vi "EventLog.Buffer.Reload.vi"(8 "error in":errorcluster, 11 "Path":path) -> (0 "error out":errorcluster, 2 "#loaded entries":i32)   [LabVIEW 2016]
uses:
  EventLog.Buffer.Action.ctl
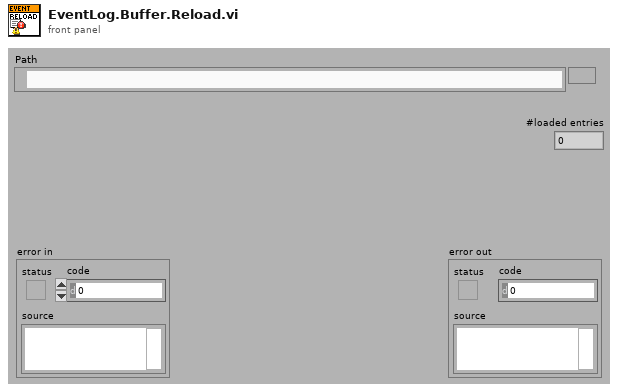
[diagram p1: front panel]
types:
  T1 = typedef "EventLog.Buffer.Action.ctl" = enum16{"init", "re-init", "clear", "set translator", "add", "get", "get unsaved"}
  T2 = typedef "EventLog.Event.ctl" = cluster{"ts":dbl, "lev":T3, "usr":i32, "src":T4, "msg":T5, "arg":variant[]}
  T3 = typedef "EventLog.EventLevel.ctl" = enum8{"Debug", "Info", "Warning", "Error"}
  T4 = typedef "EventLog.EventSource.ctl" = enum16{"All", "Gui", "Ref", "File", "Arch", "Seq", "CPX", "DB", "Laser", "Scan.P", "Scan.O", "PLC"}
  T5 = typedef "Translator.Message.ctl" = enum16{"-", "Event confirmed", "Log out", "Log in", "Shutdown", "Cancel", "Start", "Begin time", "End time", "Duration", "Service Mode", "Ignore Results", "Serial Format", "On", "Off", "OK", "NOK", "NOK %s", "Home", "Work", "Close", "Open", "In progress...", "Missing", "Empty", "Hardware failure", "Initial", "Default", "Total", "Out of range", "Free disk space is below 1GB - contact technician", "Error %d >> %s", "Error %d >> %s >> %s", "Msg %d >> %s", "Laser msg %d %s", "Laser cmd error %s %d", "Laser cmd failed %s", "Laser cmd warning %s", "Laser disconnected", "Laser status %s", "Laser already started", "Laser job unkonwn %s", "Laser job missing %s", "Laser job select failure %s", "Unable to start laser printing (%s)", "Unable to stop laser printing (%s)", "Laser marking aborted", "Laser marking timeout", "Unable to reset Laser Interlock (%s)", "Unable to trigger Laser. Laser not ready (%s)", "Laser job '%s' coordinates not configured", "Starting %s", "Quitting %s", "Configured", "Initializing", "Quitting", "Loading", "Loaded %d results", "Loaded %d events", "Running", "Stopped", "Summary", "Laser", "Do you want to continue?", "Do you want to delete the configuration?", "The configuration is being used by an order. Unable to delete!", "Press confirm button", "Station is not based. Do you want to exit?", "Station requires changeover. Do you want to run the test?", "Test options are not set as default. Do you want to continue?", "Formatting of WabcoNo is disabled. Do you want to continue?", "Product not detected. Do you want to continue?", "Product scan failed. Do you want to continue?", "Calibration", "Log out?", "System", "All", "IDLE", "Translating...%s", "Not found", "Alarm %s", "Run", "Skip", "Abort", "Repeat", "Please wait...", "Database disconnected", "Database disconnected - changeover disabled!", "Login to database successful", "Login to database failed: %d; %s", "Unable to check the product status of reference %d - database disconnected", "Unable to set the product status of reference %d - database disconnected", "Variant file backup %s", "Read variant (%s)", "Result", "Station armed!", "Station requires changeover!", "Select reference number...", "EMERGENCY BUTTON - press Control button", "EMERGENCY DOOR - press Control button", "Resetting Emergency...", "Unable to reset safety circuit - Emergency Button pressed", "Unable to reset safety circuit - Emergency Side Door open", "Station not based", "Station based", "Station not empty", "Station basing...", "No order", "Press Start to begin new order", "Scanning new order", "Order NOK. Correct or scan again", "Order OK. Press Accept", "Order ready", "Revolver incorrect", "Fork incorrect", "Revolver missing", "Revolver empty", "Container missing", "Offline results", "Offline statistics", "Updating statistics %.1f %%", "DMC Configurator", "Door open", "Close the front door", "Press start button", "Done. Open the front door", "Running...", "Running...%.1f %%", "Pause %s", "Pause %s. NOK container missing", "Pause %s. OK container missing", "Pause %s. Revolver empty", "Pause %s. Revolver missing", "Pause %s. Revolver incorrect", "Pause %s. Fork missing", "Pause %s. Fork incorrect", "Pause %s. Too many failures", "Pause %s. Unloading failure", "Pause %s. One slot is not working", "Pause %s. Part order is done. Empty OK container", "Pause %s. Unable to move product to slot", "Pause %s. Unable to move back product pusher", "Pause %s. Unable to lift product", "Pause %s. Unable to move back product lifter", "Pause %s. Unable to move product arm to Work", "Pause %s. Unable to move product arm to NOK", "Pause %s. Unable to move product arm to OK", "Pause %s. Unable to unsuck the NOK product", "Pause %s. Unable to drop the NOK product", "Pause %s. Product OK missing", "Pause %s. Unable to unsuck the OK product", "Pause %s. Unable to drop the OK product", "Stopping...", "File '%s' is missing", "File '%s' is broken", "File '%s' is running", "Log file started (%s)", "Log file ended (%s)", "Log file stopped (%s)", "Log file ignored (%s)", "Log file exported (%s)", "Log file export failed (%s)", "Wrong serial number in log file", "Wrong reference number in log file", "Test steps are missing", "%s = %.3f", "Process param '%s' not found in DB", "Process param '%s' wrong order", "Process param '%s' value %.3f out of limits (%.3f; %.3f)", "Step%d param '%s' not found in DB", "Step%d param '%s' wrong order", "Step%d param '%s' value %.3f out of limits (%.3f; %.3f)", "Step%d EV '%s' not found in DB", "Step%d EV '%s' wrong order", "\"%s\" not found in DB", "\"%s\" wrong order", "\"%s\" value %.3f out of limits (%.3f; %.3f)", "\"%s\" not found in software", "Process init (%s)", "Process started", "Process restarted", "Process run", "Process done", "Process done - remove OK container", "Process aborted", "Process aborted at work", "Process aborted at home", "Process error", "Process error at home", "Process error at work", "Process close", "Process pause", "Process continue", "Process door open", "Process door close", "Process pause at slot %s due to %s", "Select plate from the order to process", "Do you want to start the process?", "Do you want to continue the process?", "There is unfinished order. Do you want to put the new order?", "Product %s %d OK", "Product %s %d NOK", "Unable to unload the slot %s. Product missing in the slot", "Unable to unload the slot %s. Product already in the arm", "Unable to accept the product as OK. Product missing in slot %s", "Unable to accept the product as OK. Product could not drop into the container at slot %s", "Unable to accept the product as NOK. Product could not drop into the container at slot %s", "Scan failed. Error %s", "Scan failed. Scanner disconnected", "Scan failed. Wrong Wabco number %d, limit (%d,%d)", "Scan failed. Wrong serial number %d, limit (%d,%d)", "Scan failed. Wrong date %d, limit (%d,%d)", "Scan failed. Wrong product wabco number %d (expected %d)", "Scan failed. Wrong product serial number %d (expected > 0)", "Scan OK %s", "Scan failed. Unable to determine table position (%s)", "Scan failed. Timeout", "Tune failed. Scanner disconnected", "Tune failed. Timeout", "%s = %d", "%s = %d->%d", "Unable to set %s = %.2f - Air Pressure Inside off", "Unable to set digital output '%s' = %d", "Unable to activate air pressure inside - timeout", "Unable to activate air pressure inside - aborted", "Unable to switch on Air Main Valve - Air Pressure Inlet off", "Unable to switch on Air Main Valve - Door open", "Unable to switch off Air Main Valve - timeout", "Unable to switch off Air Main Valve - aborted", "Unable to rotate Table - timeout", "Unable to rotate Table - aborted", "Unable to rotate Table - Product Move not in Home position", "Unable to rotate Table - Air Pressure Inside off", "Unable to rotate Table - Product Lift A not in Home position", "Unable to rotate Table - Product Lift B not in Home position", "Unable to rotate Table - unlock before movement timeout", "Unable to rotate Table - lock after movement timeout", "Unable to move Table Lock to %s position - timeout", "Unable to move Table Lock to %s position - aborted", "Unable to move Table Lock to %s position - Air Pressure Inside off", "Unable to move Table Lock to %s position - Table not in position", "Unable to move Product Lift A to %s position - timeout", "Unable to move Product Lift B to %s position - timeout", "Unable to move Product Lift A to %s position - aborted", "Unable to move Product Lift B to %s position - aborted", "Unable to move Product Lift A to %s position - Air Pressure Inside off", "Unable to move Product Lift B to %s position - Air Pressure Inside off", "Unable to move Product Lift A to %s position - Table not locked", "Unable to move Product Lift B to %s position - Table not locked", "Unable to move Product Lift A to %s position - Product Arm not in Work position", "Unable to move Product Lift B to %s position - Product Arm not in Work position", "Unable to set Product Suction Gripper %s to %s - timeout", "Unable to set Product Suction Gripper %s to %s - aborted", "Unable to set Product Suction Gripper %s to %s - Air Pressure Inside off", "Unable to set Product Suction Gripper %s to %s - Table slot unkown", "Unable to move Product Arm to %s position - timeout", "Unable to move Product Arm to %s position - aborted", "Unable to move Product Arm to %s position - Air Pressure Inside off", "Unable to move Product Arm to %s position - Product Lift A not in Home position", "Unable to move Product Arm to %s position - Product Lift B not in Home position", "Unable to move Product to %s position - timeout", "Unable to move Product to %s position - aborted", "Unable to move Product to %s position - Air Pressure Inside off", "Unable to move Product to %s position - Table not in position"}
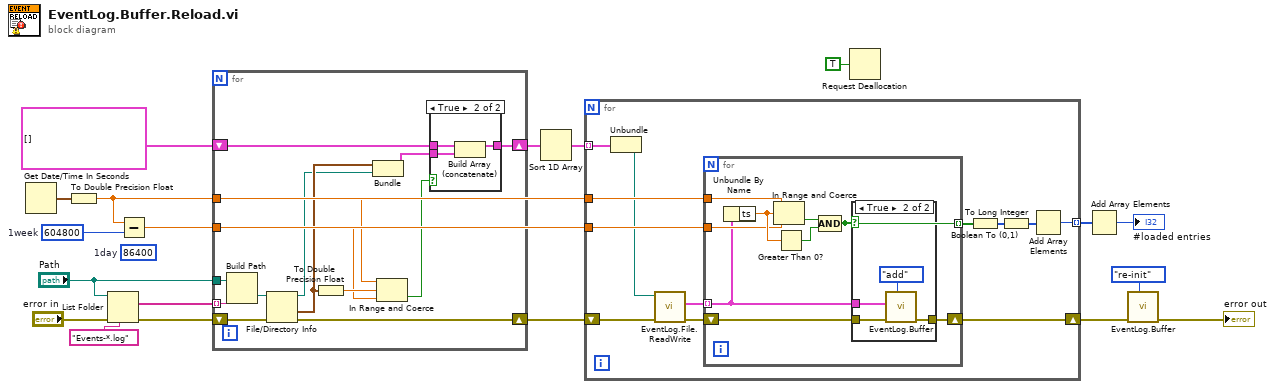
[diagram p0: block diagram]
diagram:
  w1 = 604800  # 1week
  (unwired) 86400  # 1day
  n1 = Get Date/Time In Seconds() -> (seconds since 1Jan1904=w7:timestamp)
  n2 = To Double Precision Float(number=w7) -> (double precision float=w14:dbl)
  n3 = List Folder(path="Path", pattern="Events-*.log", error in="error in") -> (filenames=w10:string[], error out=w9:errorcluster)  [unwired: 1 in, 2 out]
  n4 = Subtract(x=w14, y=w1) -> (x-y=w13:dbl)
  n5 = for {
    tunnel: "Path" -> [w22]
    tunnel: w14 -> [w24]
    tunnel: w13 -> [w23]
    shift-right: [w32] -> w17
    shift-left: cluster{"last mod":timestamp, "path out":path}[] [] ("Chart file names in use") -> [w33]
    tunnel: w10 -> [w20] mode=indexing
    shift-right: [w25] -> w16
    shift-left: w9 -> [w31]
    n6 = Build Path(base path=w22, name or relative path=w20) -> (appended path=w21:path)
    n7 = File/Directory Info(path=w21, error in=w31) -> (path out=w27:path, last mod=w28:timestamp, error out=w25:errorcluster)  [unwired: 4 out]
    n8 = To Double Precision Float(number=w28) -> (double precision float=w30:dbl)
    n9 = Bundle("last mod"=w28, "path out"=w27) -> (w26:cluster{"last mod":timestamp, "path out":path})  [unwired: 1 in]
    n10 = In Range and Coerce(upper limit=w24, x=w30, lower limit=w23) -> (In Range?=w29:bool)  [unwired: 1 out]
    n11 = case shown="True" w29 {
      tunnel: w33 -> [w34 w37]
      tunnel: [w34 w36] -> w32
      tunnel: w26 -> [_ w35]
      frame False {
      }
      frame True {
        n12 = Build Array (concatenate)(w37, w35) -> (w36:cluster{"last mod":timestamp, "path out":path}[])
      }
    }
  }
  n13 = Sort 1D Array(array=w17) -> (sorted array=w15:cluster{"last mod":timestamp, "path out":path}[])
  n14 = for {
    shift-right: [w48] -> w5
    shift-left: w16 -> [w45]
    tunnel: w15 -> [w49] mode=indexing
    tunnel: w14 -> [w47]
    tunnel: w13 -> [w46]
    tunnel: [w38] -> w3 mode=indexing
    n15 = Unbundle(w49) -> ("path out"=w42:path)  [unwired: 1 out]
    n16 = call "EventLog.File.ReadWrite.vi"("error in"=w45, "file"=w42) -> ("error out"=w44:errorcluster, "Events out"=w43:T2[])  [unwired: 5 in, 3 out]
    n17 = for {
      tunnel: w43 -> [w51] mode=indexing
      tunnel: w47 -> [w55]
      tunnel: w46 -> [w54]
      shift-right: [w52] -> w48
      shift-left: w44 -> [w53]
      tunnel: [w50] -> w41 mode=indexing
      n18 = Unbundle By Name(w51) -> ("ts"=w56:dbl)
      n19 = In Range and Coerce(upper limit=w55, x=w56, lower limit=w54) -> (In Range?=w58:bool)  [unwired: 1 out]
      n20 = Greater Than 0?(x=w56) -> (x > 0?=w57:bool)
      n21 = Compound Arithmetic op=AND(w58, w57) -> (w50:bool)
      n22 = case shown="True" w50 {
        tunnel: w53 -> [w59 w62]
        tunnel: [w59 w61] -> w52
        tunnel: w51 -> [_ w60]
        frame False {
        }
        frame True {
          n23 = call "EventLog.Buffer.vi"("action (get)"=EventLog.Buffer.Action."add" ("action (read)"), "error in"=w62, "Event in"=w60) -> ("error out"=w61:errorcluster)  [unwired: 5 in, 3 out]
        }
      }
    }
    n24 = Boolean To (0,1)(Boolean=w41) -> (0, 1=w40:i16[])
    n25 = To Long Integer(number=w40) -> (32bit integer=w39:i32[])
    n26 = Add Array Elements(numeric array=w39) -> (sum=w38:i32)
  }
  n27 = Request Deallocation(TRUE ("flag")) -> ()
  n28 = Add Array Elements(numeric array=w3) -> (sum=→"#loaded entries":i32)
  n29 = call "EventLog.Buffer.vi"("action (get)"=EventLog.Buffer.Action."re-init" ("action (read)"), "error in"=w5) -> ("error out"=→"error out":errorcluster)  [unwired: 6 in, 3 out]
